vi "3-2.vi"(10 "量化阶Δ(V)":dbl=0.02, 11 "模拟信号参数":cluster{"频率(Hz)":dbl, "幅值(V)":dbl}={"频率(Hz)"=100.0, "幅值(V)"=2.5}) -> (1 "信噪比(dB)":dbl, 2 "量化噪声":waveform(dbl)(graph), 3 "复原信号":waveform(dbl)(graph))   [LabVIEW 2018]
uses:
  <vilib>/measure/NI_MABase.lvlib
panel:
  out "噪声平均功率":dbl
  out "信号平均功率":dbl
  out "输入信号":waveform(dbl)(graph)
  # "信噪比理论值为\n49.92dB\n（L取8，幅值为2.5V）"
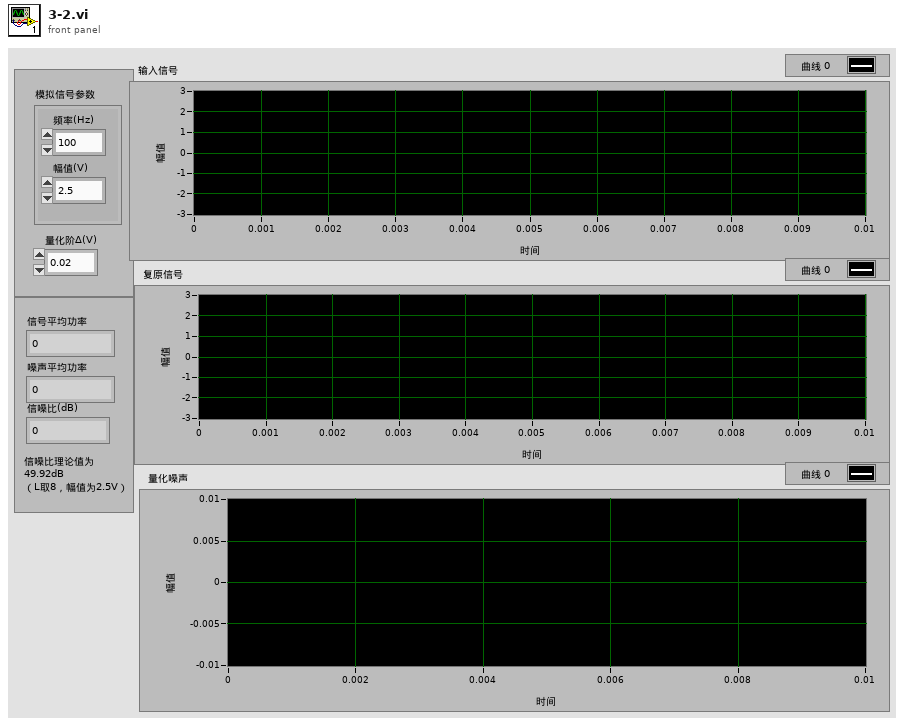
[diagram p1: front panel]
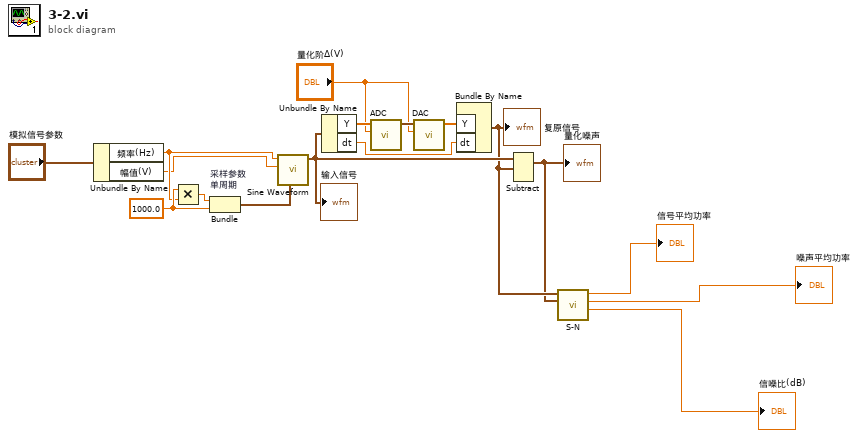
[diagram p0: block diagram]
diagram:
  w15 = 1000.0 ("x")
  n1 = Unbundle By Name("模拟信号参数") -> ("频率(Hz)"=w13:dbl, "幅值(V)"=w12:dbl)
  n2 = Multiply(x=w15, y=w13) -> (x*y=w16:dbl)
  n3 = Bundle "采样参数\n单周期"(w16, "x"=w15) -> (w14:cluster{dbl, "x":dbl})  [unwired: 1 in]
  n4 = call <vilib>:"Sine Waveform.vi"("sampling info"=w14, "amplitude"=w12, "frequency"=w13) -> ("signal out"=w6:waveform(dbl))  [unwired: 7 in, 1 out]
  "输入信号" <- w6
  n5 = Unbundle By Name(w6) -> ("Y"=w11:dbl[], "dt"=w7:dbl)
  n6 = call "ADC.vi"("量化阶Δ(V)"="量化阶Δ(V)", "信号数组(V)"=w11) -> ("编码数组"=w10:digitaldata)  [unwired: 9 in]
  n7 = call "DAC.vi"("量化阶Δ(V)"="量化阶Δ(V)", "编码信号数组"=w10) -> ("还原信号数组"=w8:dbl[])  [unwired: 9 in]
  n8 = Bundle By Name("Y"=w8, "dt"=w7) -> (w5:waveform(dbl))  [unwired: 1 in]
  "复原信号" <- w5
  n9 = Subtract(1:w5, 2:w6) -> (0:w4:waveform(dbl))  [unwired: 1 in, 1 out]
  "量化噪声" <- w4
  n10 = call "S-N.vi"("noise"=w4, "signal"=w5) -> ("信噪比(dB)"=→"信噪比(dB)":dbl, "噪声平均功率"=→"噪声平均功率":dbl, "信号平均功率"=→"信号平均功率":dbl)  [unwired: 7 in]
